vi "Wavelets Bands Explorer.vi"() -> ()   [LabVIEW 2023]
uses:
  Images/_Images.ctl
  <vilib>/vision/NI_Vision_Development_Module.lvlib
  <vilib>/addons/_Advanced Signal Processing/NI_AdvSigProcWA.lvlib
panel:
  out "Same!":bool
  out "Image 2":T1(plugin-control)
  in  "Image":T2=enum."Battery1"
  in  "Wavelet":i32(ring) items=["db02"=0, "db03"=1, "db04"=2, "db05"=3, "db06"=4, "db07"=5, "db08"=6, "db09"=7, "db10"=8, "db11"=9, "db12"=10, "db13"=11, "db14"=12, "Haar"=13, "bior1_3"=14, "bior1_5"=15, "bior2_2"=16, "bior2_4"=17, "bior2_6"=18, "bior2_8"=19, "bior3_1"=20, "bior3_3"=21, "bior3_5"=22, "bior3_7"=23, "bior3_9"=24, "bior4_4 (FBI)"=25, "bior5_5"=38, "bior6_8"=39, "coif1"=26, "coif2"=27, "coif3"=28, "coif4"=29, "coif5"=30, "sym2"=31, "sym3"=32, "sym4"=33, "sym5"=34, "sym6"=35, "sym7"=36, "sym8"=37]
  out "LLL":T1(plugin-control)
  out "LHH":T1(plugin-control)
  out "LHL":T1(plugin-control)
  out "LLH":T1(plugin-control)
  out "HH":T1(plugin-control)
  out "HL":T1(plugin-control)
  out "LH":T1(plugin-control)
  out "LL":T1(plugin-control)
  out "Image":T1(plugin-control)
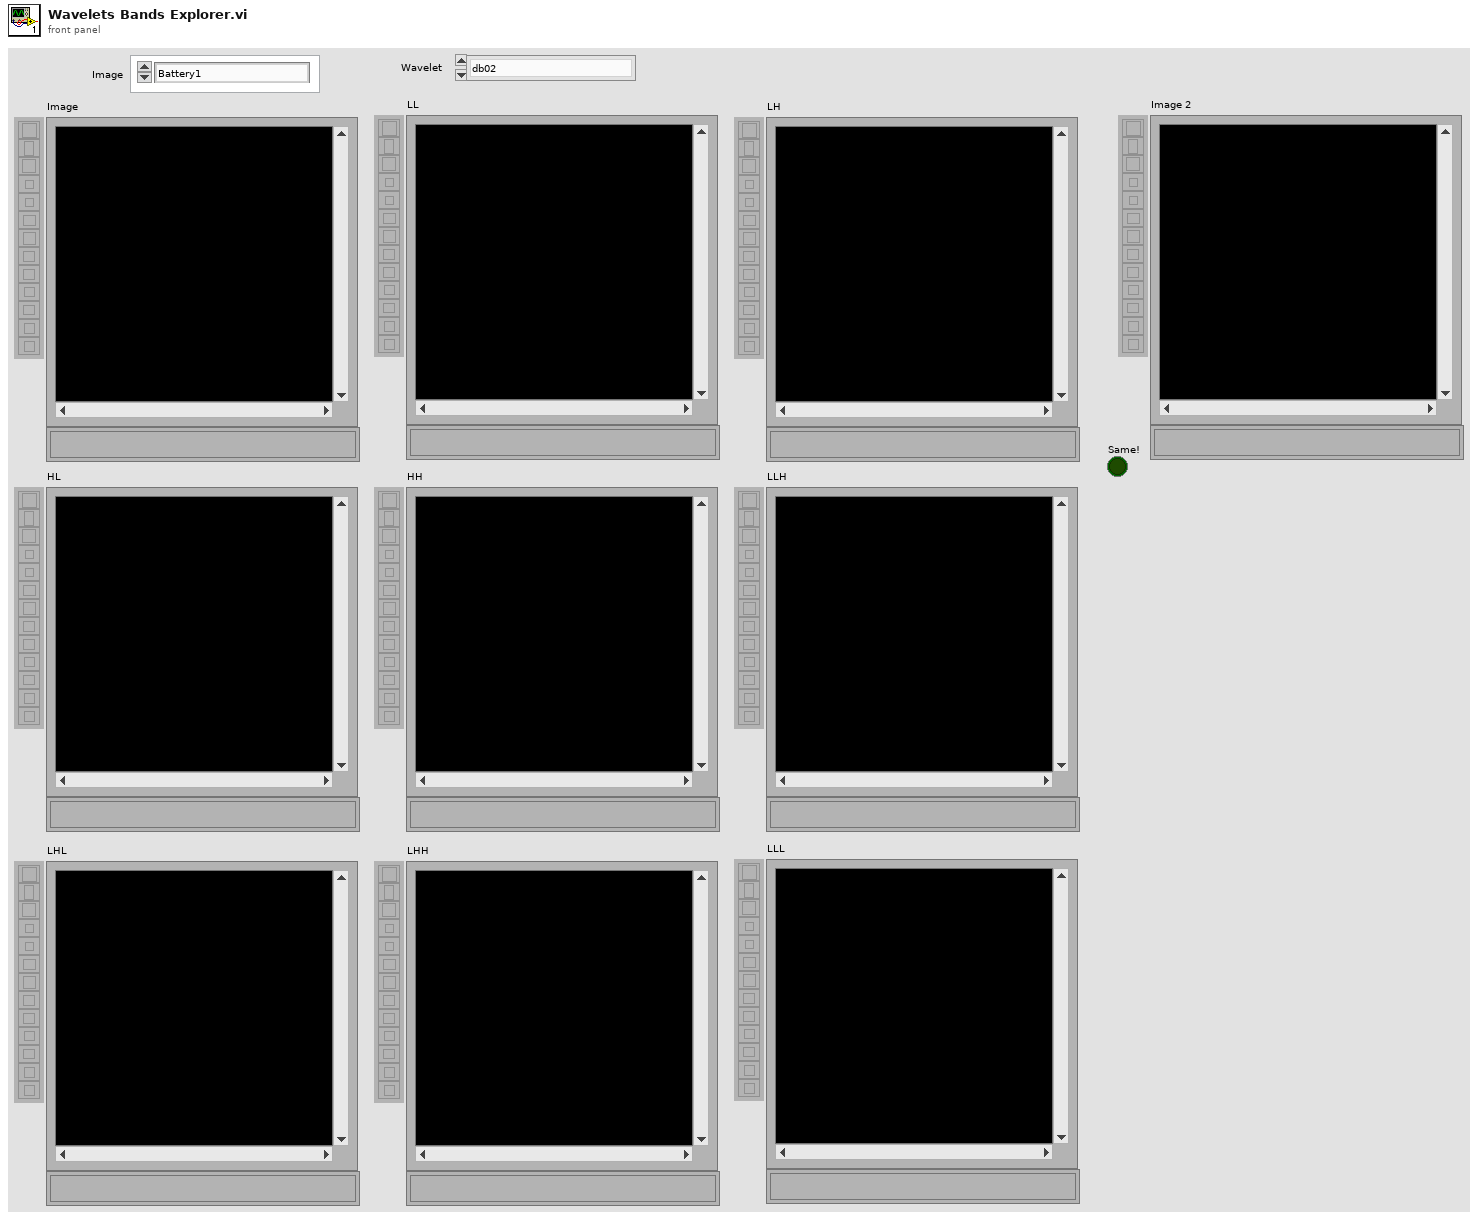
[diagram p1: front panel]
types:
  T1 = typedef "IMAQ Image.ctl" = refnum<image>
  T2 = typedef "_Images.ctl" = enum16{"Balls2", "Battery1", "Battery2", "Connector1", "Subwoofer1", "Subwoofer2", "Subwoofer3", "Subwoofer4", "Hase1", "Lamp1", "Lamp2", "Mouse1", "PhotoLens1", "Po1", "PowerSupply1", "Router", "--- Step Wedges ---", "Stepwedge1", "Stepwedge2", "Stepwedge3", "--- Fusion ---", "Fusion160kV", "Fusion2-120kV", "Fusion2-320kV", "Fusion300kV", "FusionPart1-120kV", "FusionPart1-180kV", "--- PART 01 ---", "Part1", "Part2", "Part3", "Part4", "Part5", "Part6", "Part7", "Part8", "--- Different Integrations ---", "Step2737-02Int", "Step2737-04Int", "Step2737-08Int", "Step2737-16Int", "Step2737-32Int", "Step2737-64Int"}
  T3 = typedef "Image Type" = u32
  T4 = cluster{"Type":i32, "Wavelet Bands To Use":i32[], "Min. Energy Level":sgl}
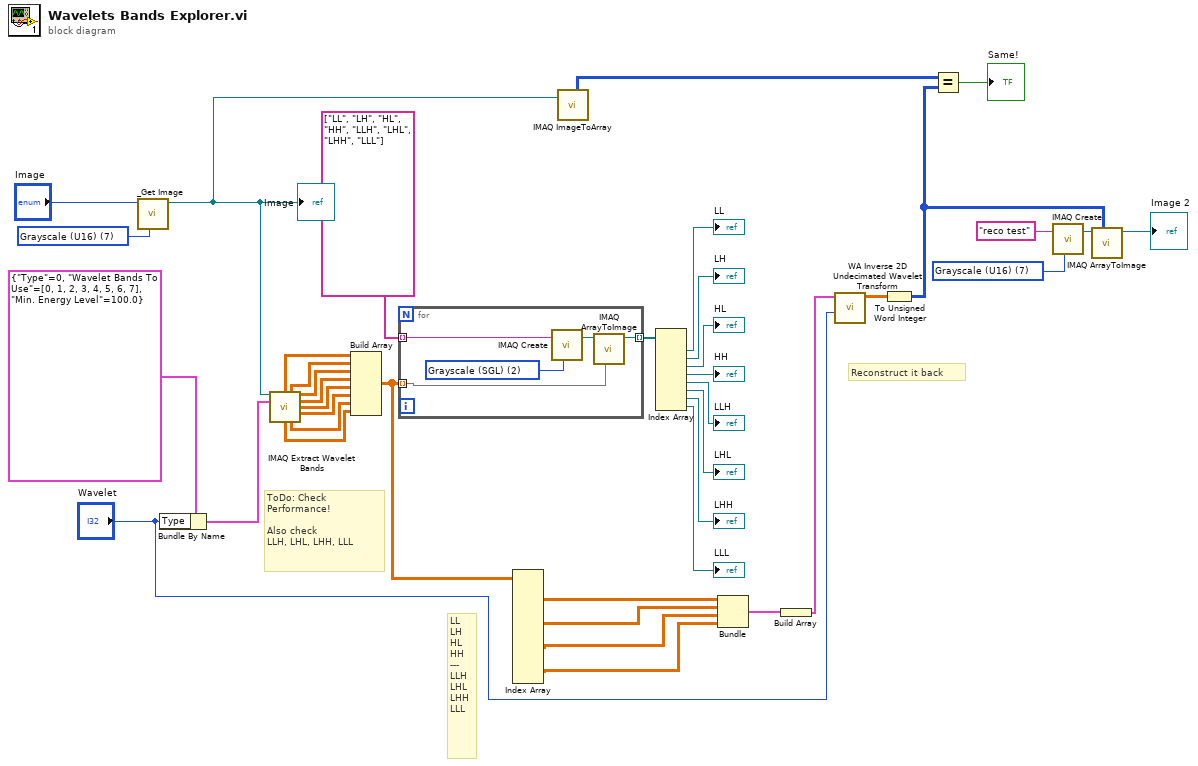
[diagram p0: block diagram]
diagram:
  w6 = T3 7 items=["Grayscale (U8)", "Grayscale (I16)", "Grayscale (SGL)", "Complex (CSG)", "RGB (U32)", "HSL (U32)", "RGB (U64)", "Grayscale (U16)"] ("Image Type (U16)")
  w15 = T3 7 items=["Grayscale (U8)", "Grayscale (I16)", "Grayscale (SGL)", "Complex (CSG)", "RGB (U32)", "HSL (U32)", "RGB (U64)", "Grayscale (U16)"] ("Image Type")
  # "ToDo: Check\nPerformance!\n\nAlso check\nLLH, LHL, LHH, LLL"
  # "Reconstruct it back"
  # "LL\nLH\nHL\nHH\n---\nLLH\nLHL\nLHH\nLLL"
  n1 = call "_Get Image.vi"("Image Type (U16)"=w6, "Image"="Image") -> ("Image Out"=w5:T1)  [unwired: 6 in, 3 out]
  "Image" <- w5
  n2 = Bundle By Name(cluster=T4 {"Type"=0, "Wavelet Bands To Use"=[0, 1, 2, 3, 4, 5, 6, 7], "Min. Energy Level"=100.0} ("Wavelet Options"), "Type"="Wavelet") -> (w19:T4)
  n3 = call "IMAQ Extract Wavelet Bands"("Image"=w5, "Wavelet Options"=w19) -> ("LL"=w38:sgl[][], "LH"=w37:sgl[][], "HL"=w36:sgl[][], "HH"=w35:sgl[][], "LLH"=w34:sgl[][], "LHL"=w33:sgl[][], "LLL"=w31:sgl[][], "LHH"=w32:sgl[][])  [unwired: 5 in, 1 out]
  n4 = Build Array(w38, w37, w36, w35, w34, w33, w32, w31) -> (w14:sgl[][][])
  n5 = for {
    tunnel: w14 -> [w41] mode=indexing
    tunnel: string[] ["LL", "LH", "HL", "HH", "LLH", "LHL", "LHH", "LLL"] -> [w44] mode=indexing
    tunnel: [w40] -> w29 mode=indexing
    w43 = T3 2 items=["Grayscale (U8)", "Grayscale (I16)", "Grayscale (SGL)", "Complex (CSG)", "RGB (U32)", "HSL (U32)", "RGB (U64)", "Grayscale (U16)"] ("Image Type")
    n6 = call "IMAQ Create"("Image Name"=w44, "Image Type"=w43) -> ("New Image"=w42:T1)  [unwired: 3 in, 1 out]
    n7 = call "IMAQ ArrayToImage"("Image Pixels (Float)"=w41, "Image"=w42) -> ("Image Out"=w40:T1)  [unwired: 8 in, 1 out]
  }
  n8 = Index Array(array=w14) -> (element #1=w13:sgl[][], element #2=w12:sgl[][], element #3=w11:sgl[][], element #4=w10:sgl[][])  [unwired: 12 in]
  n9 = call "IMAQ ImageToArray"("Image"=w5) -> ("Image Pixels (U16)"=w4:u16[][])  [unwired: 3 in, 4 out]
  n10 = Index Array(array=w29) -> (element #1=→"LL":T1, element #2=→"LH":T1, element #3=→"HL":T1, element #4=→"HH":T1, element #5=→"LLH":T1, element #6=→"LHL":T1, element #7=→"LHH":T1, element #8=→"LLL":T1)  [unwired: 8 in]
  n11 = Bundle(w13, w12, w11, w10) -> (w9:cluster{sgl[][], sgl[][], sgl[][], sgl[][]})  [unwired: 1 in]
  n12 = Build Array(w9) -> (w8:cluster{sgl[][], sgl[][], sgl[][], sgl[][]}[])
  n13 = call <vilib>:"WA Inverse 2D Undecimated Wavelet Transform.vi"("wavelet"="Wavelet", "UWT coef"=w8) -> ("signal"=w16:dbl[][])  [unwired: 2 in, 7 out]
  n14 = To Unsigned Word Integer(number=w16) -> (unsigned 16bit integer=w3:u16[][])
  n15 = Equal?(x=w4, y=w3) -> (x = y?=→"Same!":bool)
  n16 = call "IMAQ Create"("Image Name"="reco test", "Image Type"=w15) -> ("New Image"=w18:T1)  [unwired: 3 in, 1 out]
  n17 = call "IMAQ ArrayToImage"("Image Pixels (U16)"=w3, "Image"=w18) -> ("Image Out"=→"Image 2":T1)  [unwired: 8 in, 1 out]
